vi "数字时钟.vi"() -> ()   [LabVIEW 2016]
panel:
  out "时间字符串":string
  out "?":T1
  out "?":T1
  out "?":T1
  out "?":T1
  out "?":T1
  out "?":T1
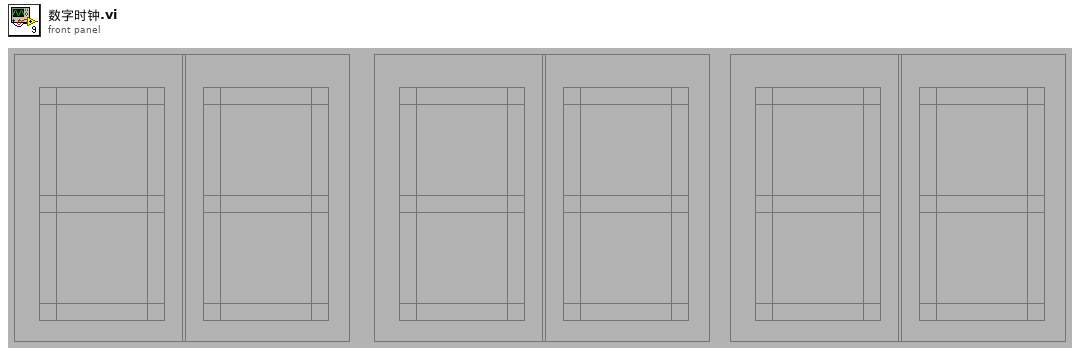
[diagram p1: front panel]
types:
  T1 = cluster{"A":bool, "D":bool, "G":bool, "B":bool, "C":bool, "F":bool, "E":bool}
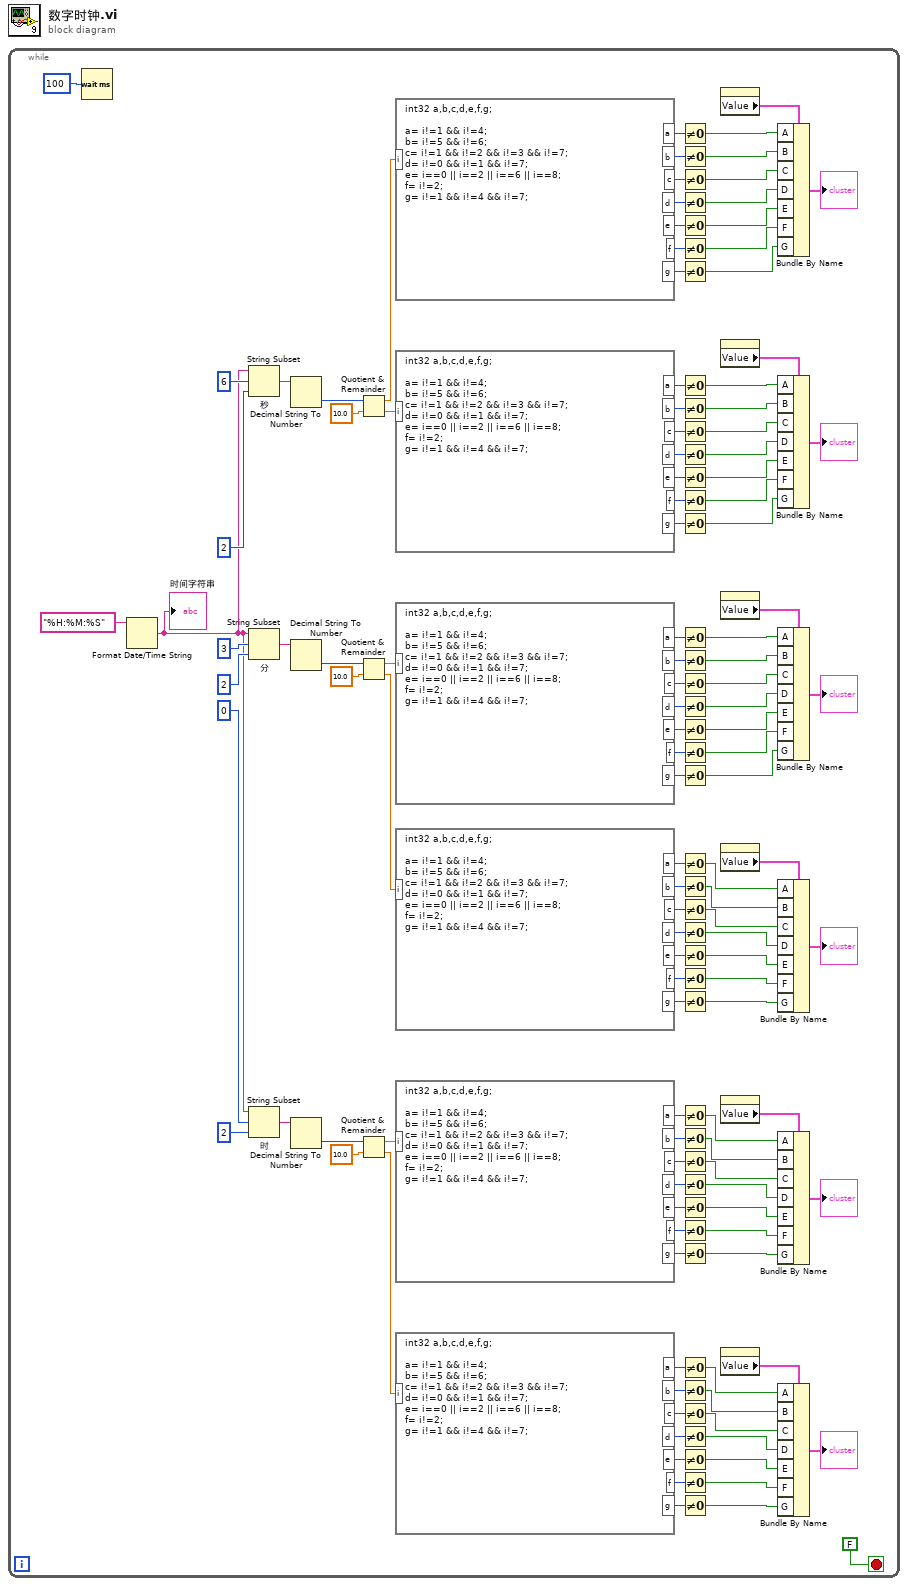
[diagram p0: block diagram]
diagram:
  n1 = while {
    stop <- FALSE stop-if-true
    n2 = Wait (ms)(milliseconds to wait=u32 100 ("等待时间（毫秒）")) -> ()  [unwired: 1 out]
    n3 = Format Date/Time String(time format string (%c)="%H:%M:%S" ("时间格式字符串(%c)")) -> (date/time string=w3:string)  [unwired: 2 in]
    "时间字符串" <- w3
    n4 = String Subset "秒"(string=w3, offset (0)=6 ("偏移量(0)"), length (rest)=2 ("长度（剩余）")) -> (substring=w7:string)
    n5 = String Subset "分"(string=w3, offset (0)=3 ("偏移量(0)"), length (rest)=2 ("长度（剩余）")) -> (substring=w1:string)
    n6 = String Subset "时"(string=w3, offset (0)=0 ("偏移量(0)"), length (rest)=2 ("长度（剩余）")) -> (substring=w12:string)
    n7 = Decimal String To Number(string=w7) -> (number=w4:i32)  [unwired: 2 in, 1 out]
    n8 = Decimal String To Number(string=w1) -> (number=w2:i32)  [unwired: 2 in, 1 out]
    n9 = Decimal String To Number(string=w12) -> (number=w13:i32)  [unwired: 2 in, 1 out]
    n10 = Quotient & Remainder(x=w4, y=10.0) -> (x-y*floor(x/y)=w45:dbl, floor(x/y)=w14:dbl)
    n11 = Quotient & Remainder(x=w2, y=10.0) -> (x-y*floor(x/y)=w52:dbl, floor(x/y)=w83:dbl)
    n12 = Quotient & Remainder(x=w13, y=10.0) -> (x-y*floor(x/y)=w118:dbl, floor(x/y)=w87:dbl)
    n13 = formula code="int32 a,b,c,d,e,f,g;\n\na= i!=1 && i!=4;\nb= i!=5 && i!=6;\nc= i!=1 && i!=2 && i!=3 && i!=7;\nd= i!=0 && i!=1 && i!=7;\ne= i==0 || i==2 || i==6 || i==8;\nf= i!=2;\ng= i!=1 && i!=4 && i!=7;"("i"=w45) -> ("a"=w44:i32, "b"=w38:i32, "c"=w37:i32, "d"=w36:i32, "e"=w35:i32, "f"=w34:i32, "g"=w33:i32)
    n14 = formula code="int32 a,b,c,d,e,f,g;\n\na= i!=1 && i!=4;\nb= i!=5 && i!=6;\nc= i!=1 && i!=2 && i!=3 && i!=7;\nd= i!=0 && i!=1 && i!=7;\ne= i==0 || i==2 || i==6 || i==8;\nf= i!=2;\ng= i!=1 && i!=4 && i!=7;"("i"=w14) -> ("a"=w29:i32, "b"=w23:i32, "c"=w22:i32, "d"=w21:i32, "e"=w20:i32, "f"=w19:i32, "g"=w18:i32)
    n15 = formula code="int32 a,b,c,d,e,f,g;\n\na= i!=1 && i!=4;\nb= i!=5 && i!=6;\nc= i!=1 && i!=2 && i!=3 && i!=7;\nd= i!=0 && i!=1 && i!=7;\ne= i==0 || i==2 || i==6 || i==8;\nf= i!=2;\ng= i!=1 && i!=4 && i!=7;"("i"=w52) -> ("a"=w53:i32, "b"=w59:i32, "c"=w60:i32, "d"=w61:i32, "e"=w62:i32, "f"=w63:i32, "g"=w64:i32)
    n16 = formula code="int32 a,b,c,d,e,f,g;\n\na= i!=1 && i!=4;\nb= i!=5 && i!=6;\nc= i!=1 && i!=2 && i!=3 && i!=7;\nd= i!=0 && i!=1 && i!=7;\ne= i==0 || i==2 || i==6 || i==8;\nf= i!=2;\ng= i!=1 && i!=4 && i!=7;"("i"=w83) -> ("a"=w68:i32, "b"=w74:i32, "c"=w75:i32, "d"=w76:i32, "e"=w77:i32, "f"=w78:i32, "g"=w79:i32)
    n17 = formula code="int32 a,b,c,d,e,f,g;\n\na= i!=1 && i!=4;\nb= i!=5 && i!=6;\nc= i!=1 && i!=2 && i!=3 && i!=7;\nd= i!=0 && i!=1 && i!=7;\ne= i==0 || i==2 || i==6 || i==8;\nf= i!=2;\ng= i!=1 && i!=4 && i!=7;"("i"=w118) -> ("a"=w117:i32, "b"=w111:i32, "c"=w110:i32, "d"=w109:i32, "e"=w108:i32, "f"=w107:i32, "g"=w106:i32)
    n18 = formula code="int32 a,b,c,d,e,f,g;\n\na= i!=1 && i!=4;\nb= i!=5 && i!=6;\nc= i!=1 && i!=2 && i!=3 && i!=7;\nd= i!=0 && i!=1 && i!=7;\ne= i==0 || i==2 || i==6 || i==8;\nf= i!=2;\ng= i!=1 && i!=4 && i!=7;"("i"=w87) -> ("a"=w102:i32, "b"=w96:i32, "c"=w95:i32, "d"=w94:i32, "e"=w93:i32, "f"=w92:i32, "g"=w91:i32)
    n19 = Not Equal To 0?(x=w44) -> (x != 0?=w43:bool)
    n20 = Not Equal To 0?(x=w38) -> (x != 0?=w42:bool)
    n21 = Not Equal To 0?(x=w37) -> (x != 0?=w41:bool)
    n22 = Not Equal To 0?(x=w36) -> (x != 0?=w40:bool)
    n23 = Not Equal To 0?(x=w35) -> (x != 0?=w39:bool)
    n24 = Not Equal To 0?(x=w34) -> (x != 0?=w31:bool)
    n25 = Not Equal To 0?(x=w33) -> (x != 0?=w32:bool)
    n26 = Not Equal To 0?(x=w29) -> (x != 0?=w28:bool)
    n27 = Not Equal To 0?(x=w23) -> (x != 0?=w27:bool)
    n28 = Not Equal To 0?(x=w22) -> (x != 0?=w26:bool)
    n29 = Not Equal To 0?(x=w21) -> (x != 0?=w25:bool)
    n30 = Not Equal To 0?(x=w20) -> (x != 0?=w24:bool)
    n31 = Not Equal To 0?(x=w19) -> (x != 0?=w16:bool)
    n32 = Not Equal To 0?(x=w18) -> (x != 0?=w17:bool)
    n33 = Not Equal To 0?(x=w53) -> (x != 0?=w54:bool)
    n34 = Not Equal To 0?(x=w59) -> (x != 0?=w55:bool)
    n35 = Not Equal To 0?(x=w60) -> (x != 0?=w56:bool)
    n36 = Not Equal To 0?(x=w61) -> (x != 0?=w57:bool)
    n37 = Not Equal To 0?(x=w62) -> (x != 0?=w58:bool)
    n38 = Not Equal To 0?(x=w63) -> (x != 0?=w66:bool)
    n39 = Not Equal To 0?(x=w64) -> (x != 0?=w65:bool)
    n40 = Not Equal To 0?(x=w68) -> (x != 0?=w69:bool)
    n41 = Not Equal To 0?(x=w74) -> (x != 0?=w70:bool)
    n42 = Not Equal To 0?(x=w75) -> (x != 0?=w71:bool)
    n43 = Not Equal To 0?(x=w76) -> (x != 0?=w72:bool)
    n44 = Not Equal To 0?(x=w77) -> (x != 0?=w73:bool)
    n45 = Not Equal To 0?(x=w78) -> (x != 0?=w81:bool)
    n46 = Not Equal To 0?(x=w79) -> (x != 0?=w80:bool)
    n47 = Not Equal To 0?(x=w117) -> (x != 0?=w116:bool)
    n48 = Not Equal To 0?(x=w111) -> (x != 0?=w115:bool)
    n49 = Not Equal To 0?(x=w110) -> (x != 0?=w114:bool)
    n50 = Not Equal To 0?(x=w109) -> (x != 0?=w113:bool)
    n51 = Not Equal To 0?(x=w108) -> (x != 0?=w112:bool)
    n52 = Not Equal To 0?(x=w107) -> (x != 0?=w104:bool)
    n53 = Not Equal To 0?(x=w106) -> (x != 0?=w105:bool)
    n54 = Not Equal To 0?(x=w102) -> (x != 0?=w101:bool)
    n55 = Not Equal To 0?(x=w96) -> (x != 0?=w100:bool)
    n56 = Not Equal To 0?(x=w95) -> (x != 0?=w99:bool)
    n57 = Not Equal To 0?(x=w94) -> (x != 0?=w98:bool)
    n58 = Not Equal To 0?(x=w93) -> (x != 0?=w97:bool)
    n59 = Not Equal To 0?(x=w92) -> (x != 0?=w89:bool)
    n60 = Not Equal To 0?(x=w91) -> (x != 0?=w90:bool)
    n61 = property class="Clust (严格)"() -> ("Value"=w47:T1)  [unwired: 2 in, 2 out]
    n62 = property class="Clust (严格)"() -> ("Value"=w15:T1)  [unwired: 2 in, 2 out]
    n63 = property class="Clust (严格)"() -> ("Value"=w50:T1)  [unwired: 2 in, 2 out]
    n64 = property class="Clust (严格)"() -> ("Value"=w82:T1)  [unwired: 2 in, 2 out]
    n65 = property class="Clust (严格)"() -> ("Value"=w120:T1)  [unwired: 2 in, 2 out]
    n66 = property class="Clust (严格)"() -> ("Value"=w88:T1)  [unwired: 2 in, 2 out]
    n67 = Bundle By Name(cluster=w47, "A"=w43, "B"=w42, "C"=w41, "D"=w40, "E"=w39, "F"=w31, "G"=w32) -> (→"?":T1)
    n68 = Bundle By Name(cluster=w15, "A"=w28, "B"=w27, "C"=w26, "D"=w25, "E"=w24, "F"=w16, "G"=w17) -> (→"?":T1)
    n69 = Bundle By Name(cluster=w50, "A"=w54, "B"=w55, "C"=w56, "D"=w57, "E"=w58, "F"=w66, "G"=w65) -> (→"?":T1)
    n70 = Bundle By Name(cluster=w82, "A"=w69, "B"=w70, "C"=w71, "D"=w72, "E"=w73, "F"=w81, "G"=w80) -> (→"?":T1)
    n71 = Bundle By Name(cluster=w120, "A"=w116, "B"=w115, "C"=w114, "D"=w113, "E"=w112, "F"=w104, "G"=w105) -> (→"?":T1)
    n72 = Bundle By Name(cluster=w88, "A"=w101, "B"=w100, "C"=w99, "D"=w98, "E"=w97, "F"=w89, "G"=w90) -> (→"?":T1)
  }
